vi "NISE.local.Open Generic Command.vi"(0 "SLSC Local in":refnum<class "SLSC Interface.lvclass">, 5 "resource":string, 7 "command in":refnum<k21>, 11 "error in (no error)":errorcluster) -> (4 "SLSC Local out":refnum<class "SLSC Interface.lvclass">, 8 "command out":refnum<k21>, 15 "error out":errorcluster)   [LabVIEW 2016, in "SLSC Interface.lvclass"]
uses:
  SLSC Interface Class/SLSC Interface.lvclass
  SLSC Interface Class/NISE.Read session.vi
  SLSC Interface Class/NISE.Write session.vi
  <vilib>/SLSC/SLSC.lvlib
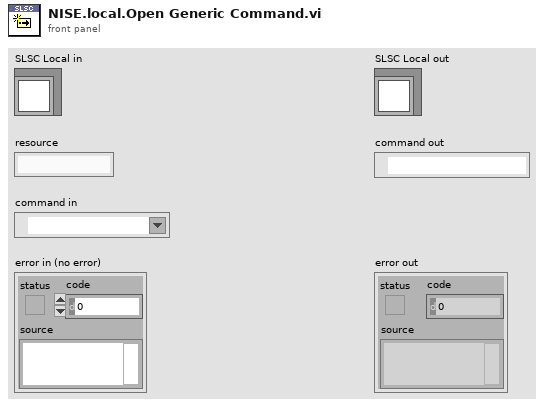
[diagram p1: front panel]
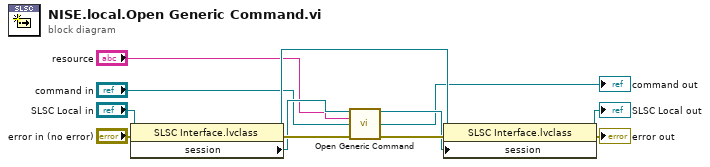
[diagram p0: block diagram]
diagram:
  n1 = property class="SLSC Interface.lvclass"(reference="SLSC Local in", error in="error in (no error)") -> (reference out=w6:refnum<class "SLSC Interface.lvclass">, error out=w11:errorcluster, "session"=w7:refnum<k21>)
  n2 = call <vilib>:"Open Generic Command.vi"("session in"=w7, "resource"="resource", "command in"="command in", "error in (no error)"=w11) -> ("session out"=w4:refnum<k21>, "command out"=→"command out":refnum<k21>, "error out"=w10:errorcluster)  [unwired: 9 in]
  n3 = property class="SLSC Interface.lvclass"(reference=w6, error in=w10, "session"=w4) -> (reference out=→"SLSC Local out":refnum<class "SLSC Interface.lvclass">, error out=→"error out":errorcluster)
